vi "scroll grafic.vi"(9 "Rango de grafica":i16, 10 "tiempo":dbl, 11 "XYGraph in":refnum<vi>) -> ()   [LabVIEW 2017]
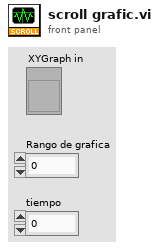
[diagram p1: front panel]
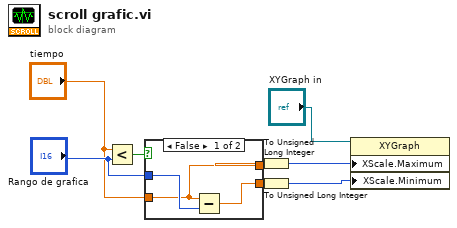
[diagram p0: block diagram]
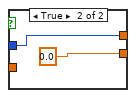
[diagram p2: hidden frame]
diagram:
  n1 = Less?(x="tiempo", y="Rango de grafica") -> (x < y?=w2:bool)
  n2 = case shown="False" w2 {
    tunnel: "Rango de grafica" -> [w10 w12]
    tunnel: [w9 w12] -> w4
    tunnel: [w11 0.0] -> w6
    tunnel: "tiempo" -> [w9 _]
    frame False {
      n3 = Subtract(x=w9, y=w10) -> (x-y=w11:dbl)
    }
    frame True {
    }
  }
  n4 = To Unsigned Long Integer(number=w4) -> (unsigned 32bit integer=w5:u32)
  n5 = To Unsigned Long Integer(number=w6) -> (unsigned 32bit integer=w7:u32)
  n6 = property on="Property Node" class="XYGraph"(reference="XYGraph in", "XScale.Maximum"=w5, "XScale.Minimum"=w7) -> ()  [unwired: 1 in, 2 out]
